vi "SGD 710 Stufe aufteilen.vi"(5 "auto Scan Points":bool, 7 "Punkte umkehren":bool, 8 "error in (no error)":errorcluster caption="Fehler (Eingang, kein Fehler)", 10 "Component Index":i32, 11 "Stufen Tabelle in":T1) -> (0 "error out":errorcluster caption="Fehler (Ausgang)", 2 "Komponente out":T2, 3 "Stufen Tabelle out":T1)   [LabVIEW 2020, in "Linearisierung v2.lvlib" / "Gasteiler.lvlib"]
uses:
  Gasteiler.lvlib
  Stufen Tabelle.ctl
  Visualisierungs Elemente/Auswahlfeld.ctl
  Aktion Lin Daten aufarbeiten.ctl
  Aktion FGV Gasteiler Korrektur.ctl
  Linearisierung v2.lvlib
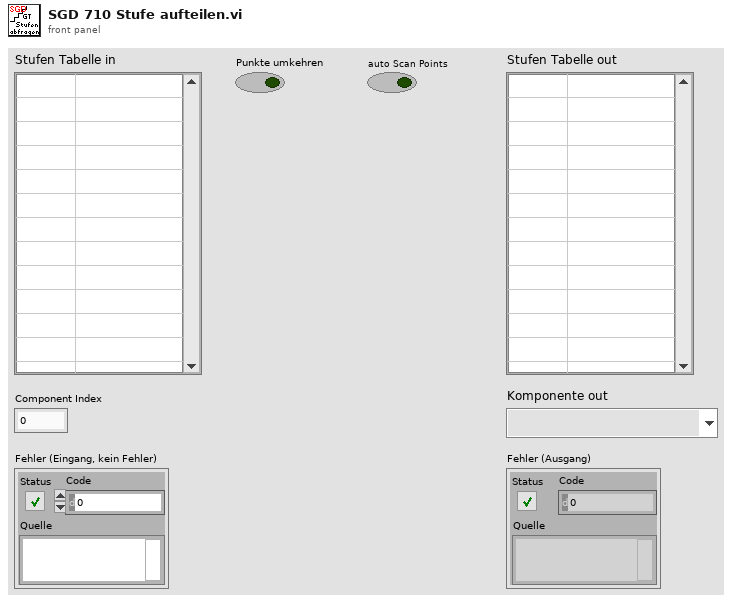
[diagram p1: front panel]
types:
  T1 = typedef "Linearisierung v2.lvlib/Gasteiler.lvlib/Stufen Tabelle.ctl" = string[][]
  T2 = typedef "Auswahlfeld.ctl" = u16
  T3 = typedef "Linearisierung v2.lvlib/Aktion Lin Daten aufarbeiten.ctl" = enum16{"lesen", "Protkolldaten", "speichern", "laden", "EPA auswerten", "Tabelle schreiben", "Lin auswerten", "Tab init", "Stufentabelle", "EPA aktiviert", "Nachbehandlung laden", "Tabelle löschen", "Istwerte löschen", "Zeile löschen", "Zeile einfügen", "LIN aktiviert", "LIN/EPA aktiv laden", "EGAK Tab"}
  T4 = typedef "Linearisierung v2.lvlib/Lin-Polynom Daten.ctl" = cluster{"Messgerät":string, "Kalibrator (Gasteiler)":string, "Bearbeiter/in":string, "Komponente":string, "Zeitstempel":timestamp, "F_max gefordert (%)":sgl, "F_max in %":sgl, "F_max in ppm":sgl, "Vorschlag Ordnung":i32, "Polynom OK":bool, "Polynomkoeff.":sgl[], "Prüfgas Konzentration":dbl, "Pfad1":string, "Pfad_LIN":string, "Gasnummer:":u8, "Komponentenauswahl":T5, "Verdünnungsgas":T6, "Zeitdauer Stufe":T7, "Anzahl Stufen":T7, "F_max in % EPA":sgl, "F_max in ppm EPA":sgl, "F_max in % LIN":sgl, "F_max in ppm LIN":sgl, "Punkte umkehren":bool, "EPA Optionsfeld":T8, "Autolin Hovacal":T9, "Span":sgl[], "Kalibrierauswahl":T10, "Conditions:":T11, "Gasflaschen Nr.:":string, "Bottle Accuracy":dbl, "Konfig Gasflasche":T12, "Gasflasche":T13, "HovaCAL Flow AutoLin":T14, "MFC Output":T15, "Gas Ablaufdatum":timestamp, "Modus":T16, "zusätzliche Zeitdauer Erster Punkt":sgl}
  T5 = typedef "Linearisierung v2.lvlib/KomponentenArray.ctl" = cluster{"Komponente:":T2, "Konzentration":dbl}[]
  T6 = typedef "Linearisierung v2.lvlib/Gasteiler.lvlib/Prüfgas in.ctl" = u16
  T7 = typedef "Zahlen-Eingabefeld.ctl" = sgl
  T8 = typedef "Linearisierung v2.lvlib/EPA Optionsfeld.ctl" = enum32{"Istwert", "Rohwert", "Linearisierter Wert"}
  T9 = typedef "Linearisierung v2.lvlib/Gasteiler.lvlib/HovaCal.lvlib/AutoLin Hovacal.ctl" = enum32{"Keine Auswahl", "Optionsauswahl 1", "Optionsauswahl 2"}
  T10 = typedef "Linearisierung v2.lvlib/Kalibrieroption.ctl" = u16
  T11 = typedef "Linearisierung v2.lvlib/Linearity verification 1065-307.lvlib/Condition.ctl" = u16
  T12 = typedef "System Einstellungen V2.lvlib/Konfig Gasflasche.ctl" = bool
  T13 = typedef "System Einstellungen V2.lvlib/Gasflasche Auswahl.ctl" = u16
  T14 = typedef "Linearisierung v2.lvlib/Gasteiler.lvlib/HovaCAL_Interface.lvlib/Controls.lvlib/Flow Einstellung.ctl" = cluster{"HovaCAL Flow Input Cluster":dbl}
  T15 = typedef "Linearisierung v2.lvlib/Gasteiler.lvlib/HovaCAL_Interface.lvlib/Controls.lvlib/Pump state.ctl" = cluster{"Run":bool}
  T16 = typedef "EPA 1065.lvlib/T90 Test 1065-308.lvlib/Modus.ctl" = u16
  T17 = typedef "Linearisierung v2.lvlib/Gasteiler.lvlib/Aktion FGV Gasteiler Korrektur.ctl" = enum16{"lesen", "schreiben", "laden", "speichern", "B-nr und Gültig", "Gasteilernr.", "Vereinzeln", "aktiv"}
  T18 = typedef "Linearisierung v2.lvlib/Eingabetabelle.ctl" = string[][]
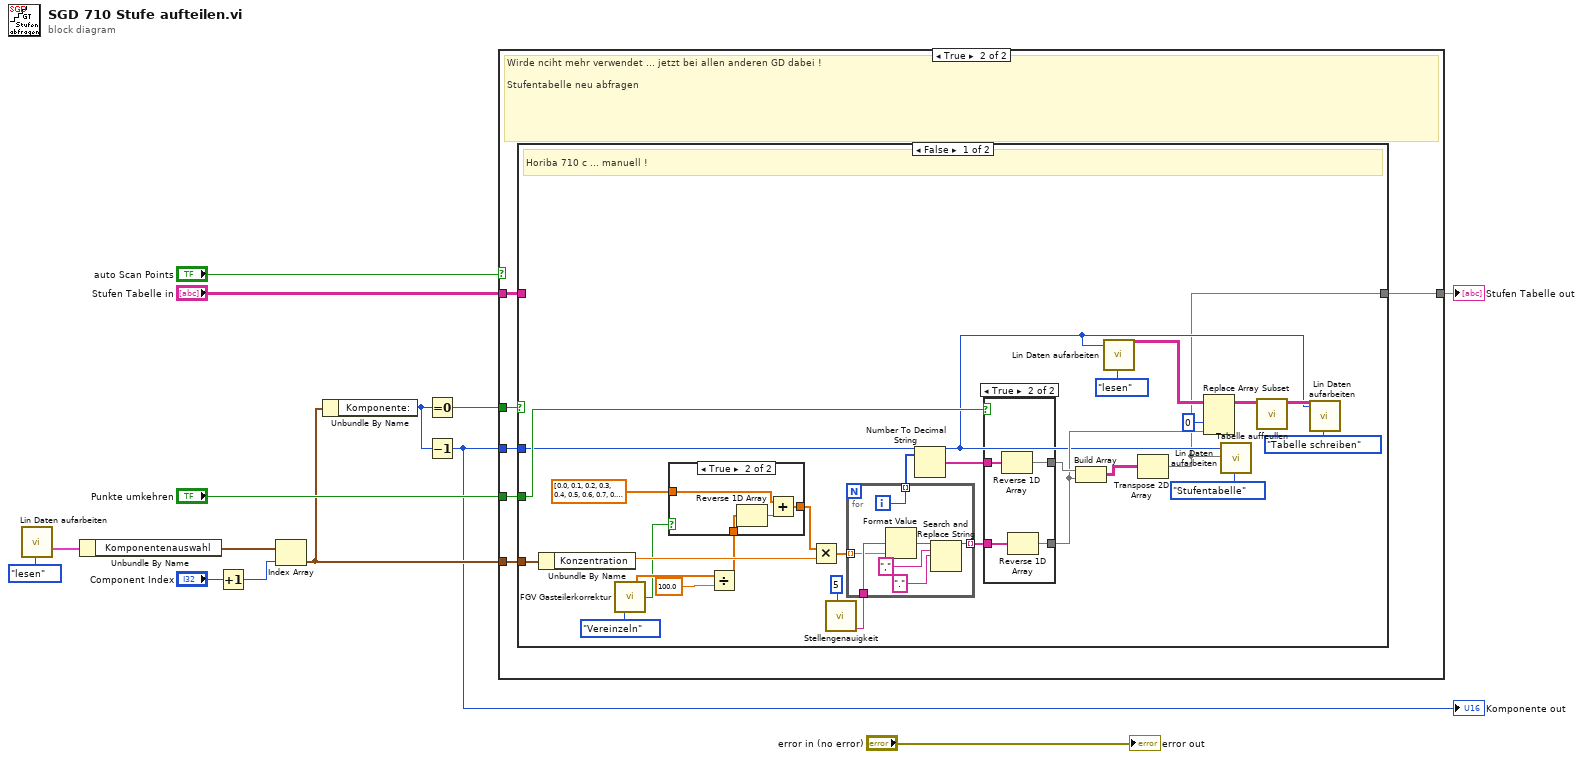
[diagram p0: block diagram]
diagram:
  n1 = call "Lin Daten aufarbeiten.vi"("Aktionen"=Aktion_Lin_Daten_aufarbeiten."lesen") -> ("Lin-Polynom"=w13:T4)  [unwired: 16 in, 10 out]
  n2 = Unbundle By Name(w13) -> ("Komponentenauswahl"=w10:T5)
  n3 = Increment(x="Component Index") -> (x+1=w7:i32)
  n4 = Index Array(array=w10, index=w7) -> (element=w8:cluster{"Komponente:":T2, "Konzentration":dbl})
  n5 = Unbundle By Name(w8) -> ("Komponente:"=w5:T2)
  n6 = Equal To 0?(x=w5) -> (x = 0?=w6:bool)
  n7 = Decrement(x=w5) -> (x-1=w4:T2)
  "Komponente out" <- w4
  n8 = case shown="True" "auto Scan Points" {
    tunnel: "Punkte umkehren" -> [_ w21]
    tunnel: w8 -> [_ w20]
    tunnel: w6 -> [_ w19]
    tunnel: w4 -> [_ w18]
    tunnel: "Stufen Tabelle in" -> [w15 w17]
    tunnel: [w15 w16] -> w1
    frame False {
      # "Stufentabelle belassen"
    }
    frame True {
      # "Wirde nciht mehr verwendet ... jetzt bei allen anderen GD dabei !\n\nStufentabelle neu abfragen"
      n9 = case shown="False" w19 {
        tunnel: w21 -> [w38 _]
        tunnel: w20 -> [w49 _]
        tunnel: w18 -> [w30 _]
        tunnel: w17 -> [_ w68]
        tunnel: [w22 w68] -> w16
        frame False {
          # "Horiba 710 c ... manuell !"
          n10 = Unbundle By Name(w49) -> ("Konzentration"=w48:dbl)
          n11 = call "FGV Gasteilerkorrektur.vi"("Aktion"=Aktion_FGV_Gasteiler_Korrektur."Vereinzeln") -> ("Vereinzelt"=w28:sgl[], "Aktiv"=w26:bool)  [unwired: 9 in, 4 out]
          n12 = Divide(x=w28, y=100.0) -> (x/y=w25:dbl[])
          n13 = case shown="True" w26 {
            tunnel: dbl[] [0.0, 0.1, 0.2, 0.3, 0.4, 0.5, 0.6, 0.7, 0.8, 0.9, 1.0] -> [w50 w54]
            tunnel: w25 -> [_ w52]
            tunnel: [w50 w53] -> w24
            frame False {
            }
            frame True {
              n14 = Reverse 1D Array(array=w52) -> (reversed array=w51:dbl[])
              n15 = Add(x=w54, y=w51) -> (x+y=w53:dbl[])
            }
          }
          n16 = Multiply(x=w24, y=w48) -> (x*y=w45:dbl[])
          n17 = call "Stellengenauigkeit.vi"("Genauigkeit (6)"=i16 5) -> ("Formatstring"=w46:string)  [unwired: 9 in, 1 out]
          n18 = for {
            tunnel: w46 -> [w67]
            tunnel: w45 -> [w66] mode=indexing
            tunnel: [w61] -> w39 mode=indexing
            tunnel: [w65] -> w43 mode=indexing
            i -> [w65]
            n19 = Format Value(format string=w67, value (0)=w66) -> (output string=w62:string)  [unwired: 1 in]
            n20 = Search and Replace String(input string=w62, search string="," ("Such-String"), replace string="." ("Ersetzungs-String (\"\")")) -> (result string=w61:string)  [unwired: 5 in, 3 out]
          }
          n21 = Number To Decimal String(number=w43) -> (decimal integer string=w41:string[])  [unwired: 1 in]
          n22 = case shown="True" w38 {
            tunnel: w41 -> [w56 w60]
            tunnel: [w56 w59] -> w40
            tunnel: w39 -> [w55 w58]
            tunnel: [w55 w57] -> w34
            frame False {
            }
            frame True {
              n23 = Reverse 1D Array(array=w60) -> (reversed array=w59:string[])
              n24 = Reverse 1D Array(array=w58) -> (reversed array=w57:string[])
            }
          }
          n25 = Build Array(w40, w34) -> (w42:string[][])
          n26 = call "Lin Daten aufarbeiten.vi"("Index (Seite)"=w30, "Aktionen"=Aktion_Lin_Daten_aufarbeiten."lesen") -> ("Eingabetabelle"=w32:T18)  [unwired: 15 in, 10 out]
          n27 = Transpose 2D Array(2D array=w42) -> (transposed array=w22:string[][])
          n28 = Replace Array Subset(array=w32, new element=w34, index (col)=0 ("Deaktivierter Index (Spalte)")) -> (w36:T18)  [unwired: 1 in]
          n29 = call "Lin Daten aufarbeiten.vi"("Index (Seite)"=w30, "Stufen Tabelle"=w22, "Aktionen"=Aktion_Lin_Daten_aufarbeiten."Stufentabelle") -> ()  [unwired: 14 in, 11 out]
          n30 = call "Tabelle auffeullen.vi"("Neue Tabelle"=w36) -> ("Tabelle"=w37:string[][])  [unwired: 10 in]
          n31 = call "Lin Daten aufarbeiten.vi"("Eingabetabelle"=w37, "Index (Seite)"=w30, "Aktionen"=Aktion_Lin_Daten_aufarbeiten."Tabelle schreiben") -> ()  [unwired: 14 in, 11 out]
        }
        frame True {
          # "Wenn 0 (----) kommt dann nicht abfragen"
        }
      }
    }
  }
  "Stufen Tabelle out" <- w1
  "error out" <- "error in (no error)"
